vi "Pendulum start Timer.vi"   [LabVIEW 2014, in "pendulumApp.lvlib"]
doc: "OOTB_API void Pendulum_startTimer();"
uses:
  pendulumApp.lvlib
  pendulumApp.dll
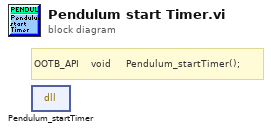
[diagram p0: block diagram]
diagram:
  # "OOTB_API    void     Pendulum_startTimer();"
  n1 = dll-call lib="E:/OneDrive - martint2560@gmail.com/code/SADI_Pendulum/LV/SADI_Pendulum_lib/pendulumApp.*" fn="Pendulum_startTimer"() -> ()  [unwired: 4 in, 2 out]
